vi "connectToMetroMini.vi"(8 "error in":errorcluster, 11 "visaName":string) -> (0 "error out":errorcluster, 2 "connected?":bool, 3 "connectedToInstrument":refnum<visa-resource-name>)   [LabVIEW 2015]
uses:
  <vilib>/Instr/_visa.llb/VISA Configure Serial Port (Instr).vi
  <userlib>/_OpenG.lib/string/string.llb/Trim Whitespace (String)__ogtk.vi
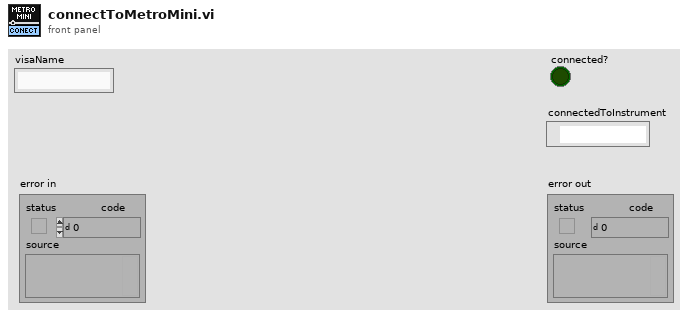
[diagram p1: front panel]
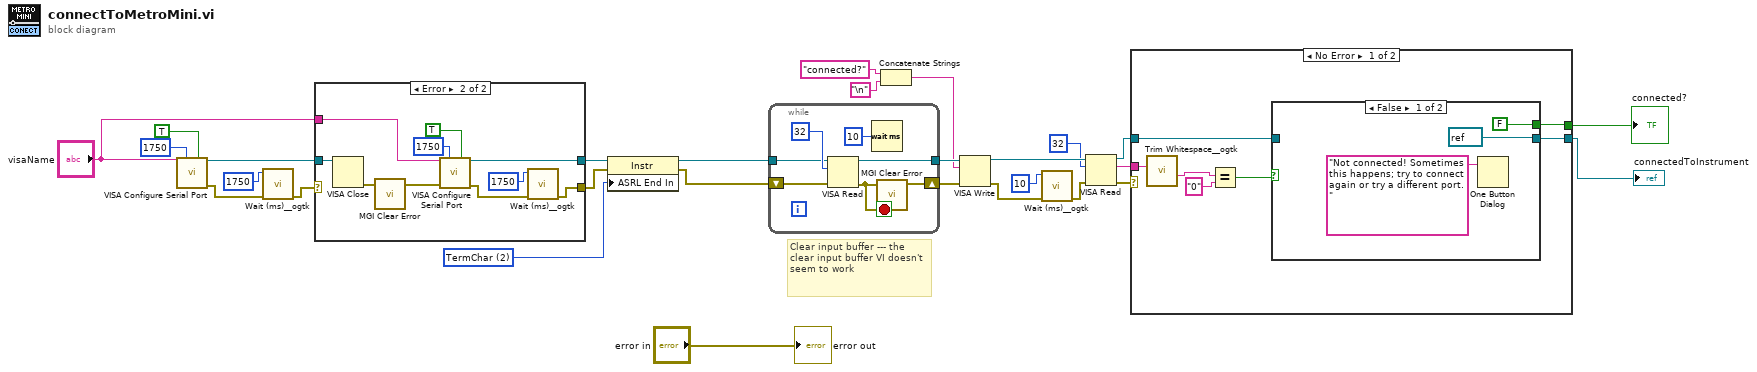
[diagram p0: block diagram]
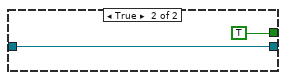
[diagram p2: hidden frame]
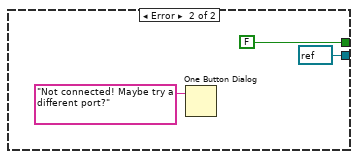
[diagram p3: hidden frame]
diagram:
  w12 = u16 2 items=["None", "Last Bit", "TermChar"] ("Serial Settings:End Mode for Reads")
  # "Clear input buffer --- the  clear input buffer VI doesn't seem to work"
  n1 = call-poly "VISA Configure Serial Port"("VISA resource name"="visaName", "timeout (10sec)"=u32 1750, "Enable Termination\nChar (T)"=TRUE ("Enable Termination\nChar (T)")) -> ("VISA resource name out"=w15:refnum<visa-resource-name>, "error out"=w13:errorcluster)  [unwired: 11 in]
  n2 = call <userlib>:"Wait (ms)__ogtk.vi"("error in (no error)"=w13, "milliseconds to wait"=u32 1750) -> ("error out"=w14:errorcluster)  [unwired: 8 in, 1 out]
  n3 = case shown="Error" w14 {
    selector: w14 -> [w29 _]
    tunnel: w15 -> [w30 w40]
    tunnel: "visaName" -> [_ w37]
    tunnel: [w29 w34] -> w18
    tunnel: [w30 w33] -> w17
    frame No Error {
    }
    frame Error {
      n4 = VISA Close(VISA resource name=w40) -> (error out=w31:errorcluster)  [unwired: 1 in]
      n5 = call <userlib>:"MGI Clear Error.vi"("Error In"=w31) -> ("Error Out"=w32:errorcluster)  [unwired: 6 in]
      n6 = call-poly "VISA Configure Serial Port"("VISA resource name"=w37, "timeout (10sec)"=u32 1750, "Enable Termination\nChar (T)"=TRUE ("Enable Termination\nChar (T)"), "error in (no error)"=w32) -> ("VISA resource name out"=w33:refnum<visa-resource-name>, "error out"=w35:errorcluster)  [unwired: 10 in]
      n7 = call <userlib>:"Wait (ms)__ogtk.vi"("error in (no error)"=w35, "milliseconds to wait"=u32 1750) -> ("error out"=w34:errorcluster)  [unwired: 8 in, 1 out]
    }
  }
  n8 = property class="Instr"(reference=w17, error in=w18, "ASRL End In"=w12) -> (reference out=w24:refnum<visa-resource-name>, error out=w1:errorcluster)
  n9 = while {
    shift-right: [w41] -> w26
    shift-left: w1 -> [w45]
    tunnel: w24 -> [w44]
    tunnel: [w43] -> w25
    stop <- w42 stop-if-true
    n10 = VISA Read(VISA resource name=w44, byte count=u32 32, error in (no error)=w45) -> (VISA resource name out=w43:refnum<visa-resource-name>, error out=w42:errorcluster)  [unwired: 2 out]
    n11 = Wait (ms)(milliseconds to wait=u32 10) -> ()  [unwired: 1 out]
    n12 = call <userlib>:"MGI Clear Error.vi"("Error In"=w42) -> ("Error Out"=w41:errorcluster)  [unwired: 6 in]
  }
  n13 = Concatenate Strings("connected?" ("write buffer"), "\n") -> (w9:string)
  n14 = VISA Write(VISA resource name=w25, write buffer=w9, error in (no error)=w26) -> (VISA resource name out=w23:refnum<visa-resource-name>, error out=w20:errorcluster)  [unwired: 1 out]
  n15 = call <userlib>:"Wait (ms)__ogtk.vi"("error in (no error)"=w20, "milliseconds to wait"=u32 10) -> ("error out"=w22:errorcluster)  [unwired: 8 in, 1 out]
  n16 = VISA Read(VISA resource name=w23, byte count=u32 32, error in (no error)=w22) -> (VISA resource name out=w4:refnum<visa-resource-name>, read buffer=w28:string, error out=w27:errorcluster)  [unwired: 1 out]
  n17 = case shown="No Error" w27 {
    tunnel: w28 -> [w54 _]
    tunnel: [w53 FALSE] -> w5
    tunnel: w4 -> [w52 _]
    tunnel: [w51 refnum<visa-resource-name> refnum ("VISA resource name out")] -> w3
    frame No Error {
      n18 = call-poly <userlib>:"Trim Whitespace__ogtk.vi"("String in"=w54) -> ("String out"=w50:string)  [unwired: 6 in]
      n19 = Equal?(x=w50, y="0" ("regular expression")) -> (x = y?=w48:bool)
      n20 = case shown="False" w48 {
        tunnel: [FALSE TRUE] -> w53
        tunnel: w52 -> [_ w58]
        tunnel: [refnum<visa-resource-name> refnum ("VISA resource name out") w58] -> w51
        frame False {
          n21 = One Button Dialog(message="Not connected! Sometimes this happens; try to connect again or try a different port.") -> ()  [unwired: 1 in, 1 out]
        }
        frame True {
        }
      }
    }
    frame Error {
      n22 = One Button Dialog(message="Not connected! Maybe try a different port?") -> ()  [unwired: 1 in, 1 out]
    }
  }
  "connectedToInstrument" <- w3
  "connected?" <- w5
  "error out" <- "error in"
